vi "StopSignal-TestMain6.vi"() -> ()   [LabVIEW 2019]
uses:
  StopSignal.lvlib
panel:
  out "error out":errorcluster
  out "reason #4":string
  out "timestamp #4":timestamp
  out "reason #3":string
  out "timestamp #3":timestamp
  out "reason #2":string
  out "timestamp #2":timestamp
  in  "stop":bool
  out "reason #1":string
  out "timestamp #1":timestamp
  out "current time":timestamp
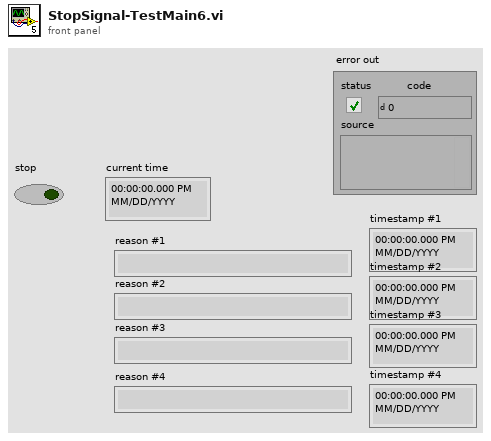
[diagram p1: front panel]
types:
  T1 = typedef "StopSignal.lvlib/StopSignal.ctl" = refnum<k1>
  T2 = typedef "StopSignal.lvlib/def-StopReason.ctl" = cluster{"Reason":string, "timestamp":timestamp}
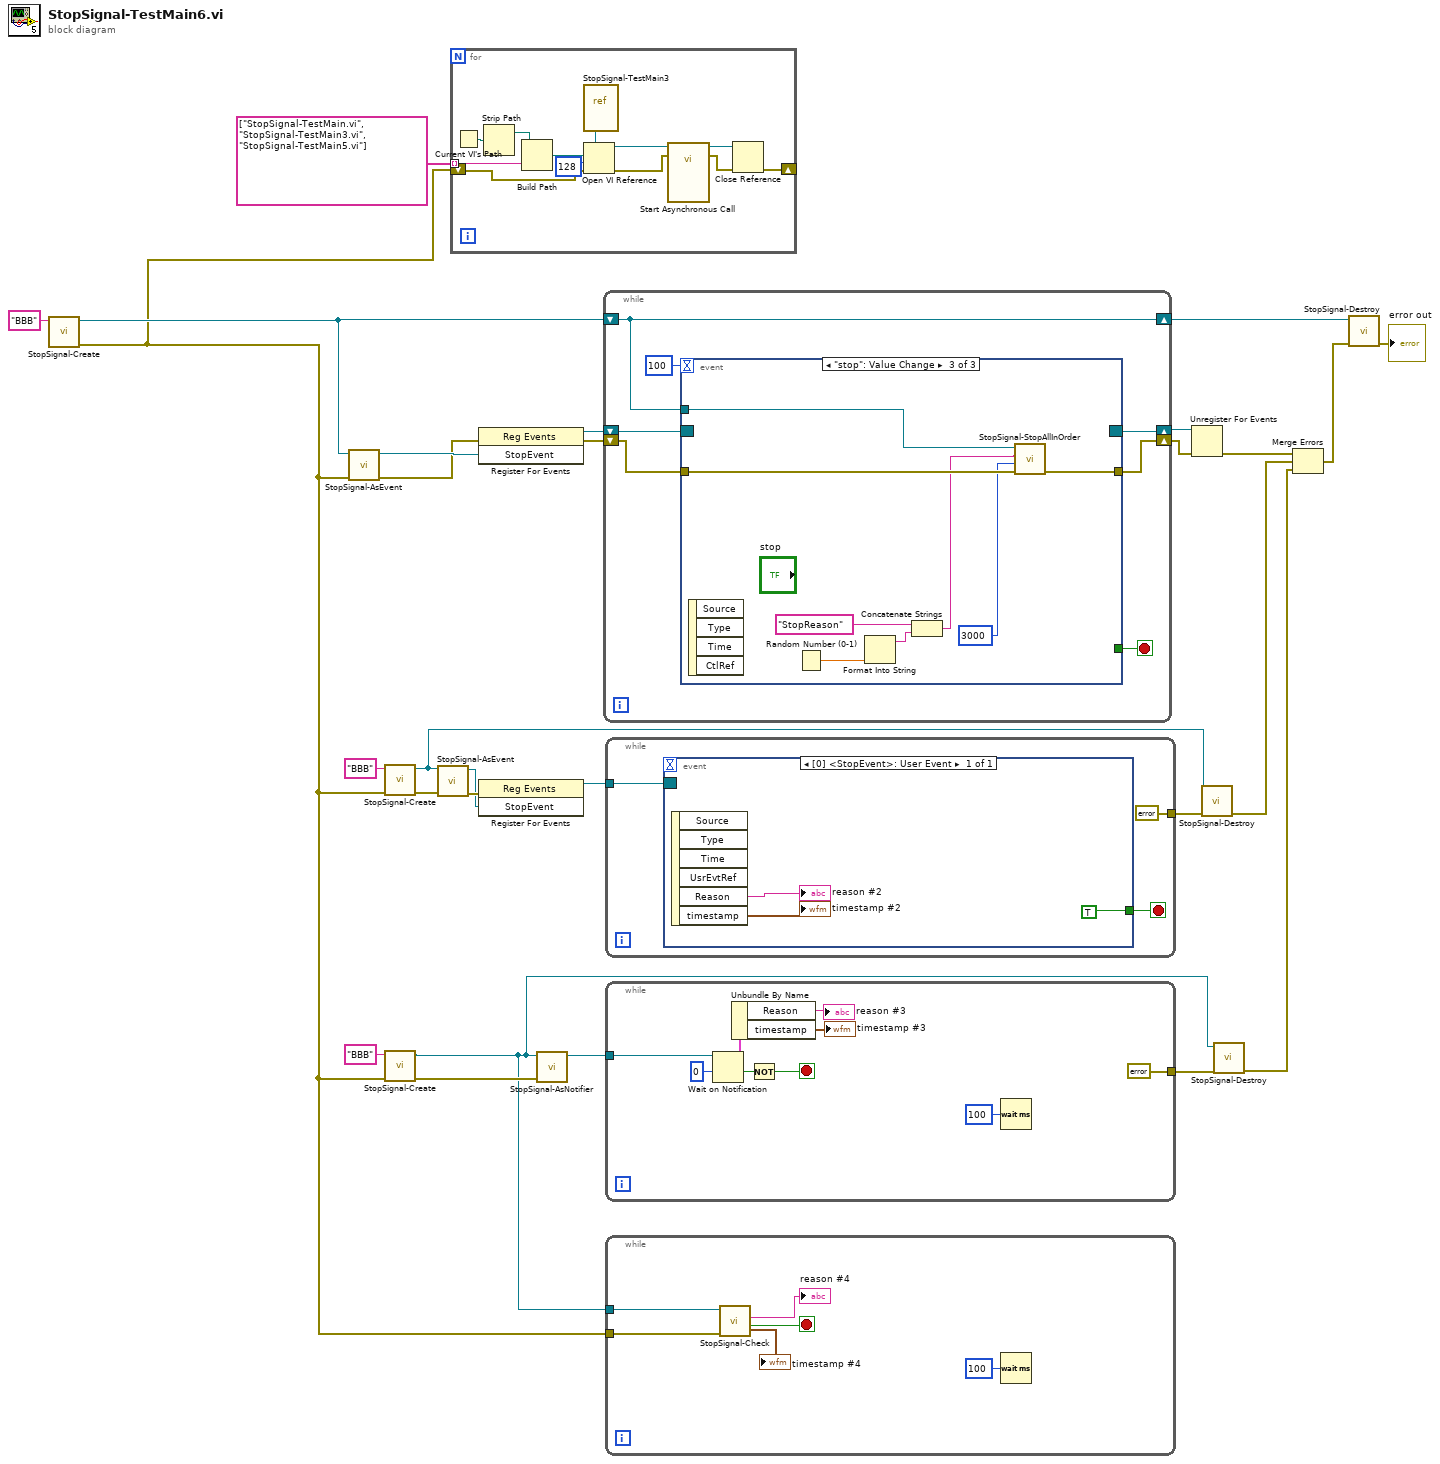
[diagram p0: block diagram]
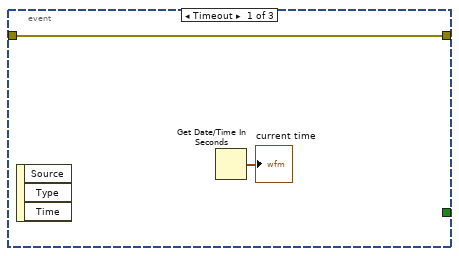
[diagram p2: hidden frame]
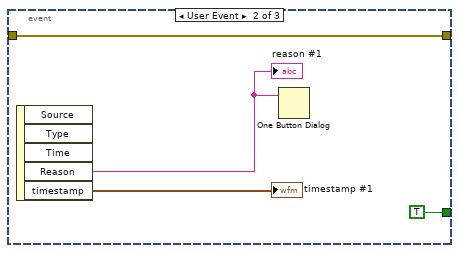
[diagram p3: hidden frame]
diagram:
  n1 = call "StopSignal-Create.vi"("name(\"\")"="BBB" ("name(\"\")")) -> ("error out"=w1:errorcluster, "StopSignal"=w21:T1)  [unwired: 8 in, 1 out]
  n2 = call "StopSignal-AsEvent.vi"("error in (no error)"=w1, "StopSignal"=w21) -> ("error out"=w6:errorcluster, "StopEvent"=w24:refnum<user-event>)  [unwired: 8 in]
  n3 = call "StopSignal-Create.vi"("error in (no error)"=w1, "name(\"\")"="BBB" ("name(\"\")")) -> ("error out"=w18:errorcluster, "StopSignal"=w15:T1)  [unwired: 7 in, 1 out]
  n4 = call "StopSignal-Create.vi"("error in (no error)"=w1, "name(\"\")"="BBB" ("name(\"\")")) -> ("error out"=w12:errorcluster, "StopSignal"=w11:T1)  [unwired: 7 in, 1 out]
  n5 = call "StopSignal-AsEvent.vi"("error in (no error)"=w18, "StopSignal"=w15) -> ("error out"=w17:errorcluster, "StopEvent"=w16:refnum<user-event>)  [unwired: 8 in]
  n6 = for {
    tunnel: string[] ["StopSignal-TestMain.vi", "StopSignal-TestMain3.vi", "StopSignal-TestMain5.vi"] -> [w39] mode=indexing
    shift-right: [w32] -> _
    shift-left: w1 -> [w31]
    n7 = Current VI's Path() -> (path=w30:path)
    n8 = Strip Path(path=w30) -> (stripped path=w29:path)  [unwired: 1 out]
    n9 = Build Path(base path=w29, name or relative path=w39) -> (appended path=w38:path)
    n10 = vi-ref "StopSignal-TestMain3.vi"() -> (w40:refnum<vi>)
    n11 = Open VI Reference(type specifier VI Refnum (for type only)=w40, vi path=w38, options=128, error in (no error)=w31) -> (vi reference=w36:refnum<vi>, error out=w35:errorcluster)  [unwired: 2 in]
    n12 = call-by-ref "Start Asynchronous Call"(reference=w36, error in=w35) -> (reference out=w33:refnum<vi>, error out=w34:errorcluster)  [unwired: 12 in]
    n13 = Close Reference(reference=w33, error in (no error)=w34) -> (error out=w32:errorcluster)
  }
  n14 = register-events(error in=w6, w24) -> (reference out=w28:refnum<event-registration>, error out=w5:errorcluster)  [unwired: 1 in]
  n15 = register-events(error in=w17, w16) -> (reference out=w26:refnum<event-registration>)  [unwired: 1 in, 1 out]
  n16 = call "StopSignal-AsNotifier.vi"("error in (no error)"=w12, "StopSignal"=w11) -> ("StopNotifier"=w22:refnum<notifier>)  [unwired: 8 in, 1 out]
  n17 = while {
    shift-right: [w44] -> w27
    shift-left: w28 -> [w47]
    shift-right: [w43] -> w23
    shift-left: w21 -> [w43]
    shift-right: [w41] -> w4
    shift-left: w5 -> [w42]
    stop <- w46 stop-if-true
    n18 = event shown="[2] \"stop\": Value Change" {
      selector: w47 -> [_ _ _]
      dyn-events: [_ _ _] -> w44
      timeout: 100 -> [_ _ _]
      tunnel: [_ TRUE _] -> w46
      tunnel: w43 -> [_ _ w54]
      tunnel: w42 -> [w48 w50 w58]
      tunnel: [w48 w50 w57] -> w41
      event Timeout {
        n19 = event-data() -> ()  [unwired: 1 in, 3 out]
        n20 = Get Date/Time In Seconds() -> (seconds since 1Jan1904=→"current time":timestamp)
      }
      event User Event {
        n21 = event-data() -> ("Reason"=w52:string, "timestamp"=→"timestamp #1":timestamp)  [unwired: 1 in, 3 out]
        "reason #1" <- w52
        n22 = One Button Dialog(message=w52) -> ()  [unwired: 1 in, 1 out]
      }
      event "stop": Value Change {
        n23 = event-data() -> ()  [unwired: 1 in, 4 out]
        n24 = Random Number (0-1)() -> (number: 0 to 1=w60:dbl)
        n25 = Format Into String(w60) -> (resulting string=w59:string)  [unwired: 3 in, 1 out]
        n26 = Concatenate Strings("StopReason" ("event data"), w59) -> (w56:string)
        n27 = call "StopSignal-StopAllInOrder.vi"("error in (no error)"=w58, "timeout(ms)"=u32 3000 ("interval time(ms)"), "reason(\"\")"=w56, "StopSignal"=w54) -> ("error out"=w57:errorcluster)  [unwired: 6 in, 1 out]
      }
    }
  }
  n28 = while {
    tunnel: w26 -> [w64]
    tunnel: [errorcluster {"status"=FALSE, "code"=0, "source"=""} ("error out")] -> w14
    stop <- w63 stop-if-true
    n29 = event shown="[0] <StopEvent>: User Event" {
      selector: w64 -> [_]
      dyn-events: _ -> [_]
      timeout: _ -> [_]
      tunnel: [TRUE] -> w63
      event User Event {
        n30 = event-data() -> ("Reason"=→"reason #2":string, "timestamp"=→"timestamp #2":timestamp)  [unwired: 1 in, 4 out]
      }
    }
  }
  n31 = while {
    tunnel: w22 -> [w72]
    tunnel: [errorcluster {"status"=FALSE, "code"=0, "source"=""} ("error out")] -> w10
    stop <- w73 stop-if-true
    n32 = Wait on Notification(notifier=w72, timeout in ms (-1)=0) -> (notification=w71:T2, timed out?=w75:bool)  [unwired: 2 in, 2 out]
    n33 = Unbundle By Name(w71) -> ("Reason"=→"reason #3":string, "timestamp"=→"timestamp #3":timestamp)
    n34 = Not(x=w75) -> (.not. x?=w73:bool)
    n35 = Wait (ms)(milliseconds to wait=u32 100) -> ()  [unwired: 1 out]
  }
  n36 = while {
    tunnel: w11 -> [w81]
    tunnel: w1 -> [w80]
    stop <- w79 stop-if-true
    n37 = call "StopSignal-Check.vi"("error in (no error)"=w80, "StopSignal"=w81) -> ("Stop?"=w79:bool, "Reason"=→"reason #4":string, "timestamp"=→"timestamp #4":timestamp)  [unwired: 5 in, 2 out]
    n38 = Wait (ms)(milliseconds to wait=u32 100) -> ()  [unwired: 1 out]
  }
  n39 = Unregister For Events(event registration refnum=w27, error in=w4) -> (error out=w25:errorcluster)
  n40 = call "StopSignal-Destroy.vi"("error in (no error)"=w14, "StopSignal"=w15) -> ("error out"=w8:errorcluster)  [unwired: 8 in, 1 out]
  n41 = call "StopSignal-Destroy.vi"("error in (no error)"=w10, "StopSignal"=w11) -> ("error out"=w7:errorcluster)  [unwired: 8 in, 1 out]
  n42 = Merge Errors(w25, w8, w7) -> (w9:errorcluster)
  n43 = call "StopSignal-Destroy.vi"("error in (no error)"=w9, "StopSignal"=w23) -> ("error out"=→"error out":errorcluster)  [unwired: 8 in, 1 out]
